vi "Set Buffer and Get Channel Reading.vi"(8 "error in":errorcluster, 9 "Readings":dbl[][](array[numeric]), 10 "Channel Ident":string, 11 "BufferLastReadingsDBL in":refnum<class "BufferLastReadsDBL.lvclass">) -> (0 "error out":errorcluster, 2 "Reading":dbl, 3 "BufferLastReadingsDBL out":refnum<class "BufferLastReadsDBL.lvclass">)   [LabVIEW 2023, in "BufferLastReadsDBL.lvclass"]
uses:
  BufferLastReadsDBL.lvclass
  BufferLastReadsDBL.lvclass/BufferLastReadsDBL.ctl
  <vilib>/Analysis/baseanly.llb/Mean (DBL).vi
  <vilib>/Analysis/NI_AALBase.lvlib
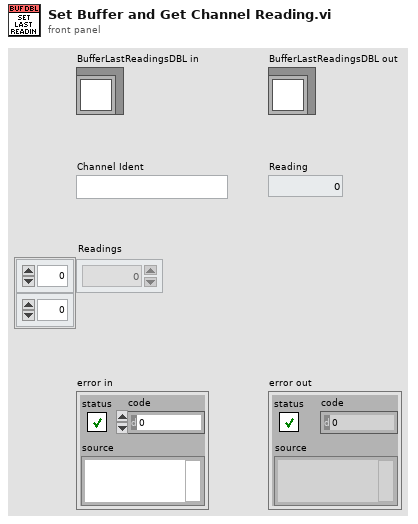
[diagram p1: front panel]
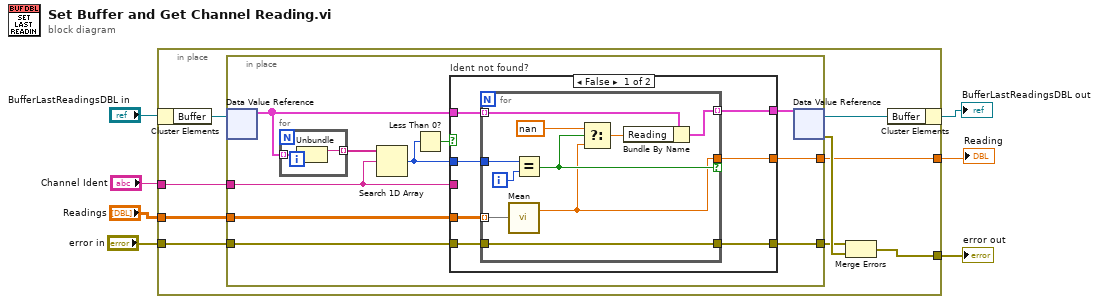
[diagram p0: block diagram]
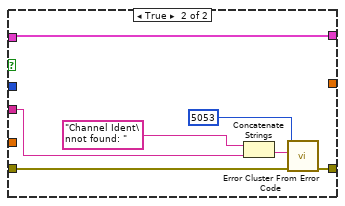
[diagram p2: hidden frame]
diagram:
  n1 = in-place {
    in-place-border: "Readings" -> [w15]
    in-place-border: "error in" -> [w14]
    in-place-border: [w12] -> w5
    in-place-border: "Channel Ident" -> [w10]
    in-place-border: [w8] -> w1
    n2 = in-place-cluster #1("BufferLastReadingsDBL in") -> ("Buffer"=w16:refnum<data-value>)
    n3 = in-place {
      in-place-border: w15 -> [w25]
      in-place-border: w14 -> [w26]
      in-place-border: w10 -> [w19]
      in-place-border: [w18] -> w9
      in-place-border: [w17] -> w8
      n4 = in-place-dvr #2(w16) -> (w21:cluster{"Ident":string, "Reading":dbl}[])  [unwired: 1 out]
      n5 = for {
        tunnel: w21 -> [w52] mode=indexing
        tunnel: [w51] -> w24 mode=indexing
        n6 = Unbundle(w52) -> ("Ident"=w51:string)  [unwired: 1 out]
      }
      n7 = Search 1D Array(1D array=w24, element=w19) -> (index of element=w22:i32)  [unwired: 1 in]
      n8 = Less Than 0?(x=w22) -> (x < 0?=w23:bool)
      n9 = case "Ident not found?" shown="False" w23 {
        tunnel: w26 -> [w28 w50]
        tunnel: w25 -> [w33 _]
        tunnel: w22 -> [w30 _]
        tunnel: w21 -> [w32 w44]
        tunnel: [w31 w44] -> w20
        tunnel: w19 -> [_ w46]
        tunnel: [w27 w45] -> w18
        tunnel: [w29 _] -> w17
        frame False {
          n10 = for {
            tunnel: w33 -> [w43] mode=indexing
            tunnel: w32 -> [w42] mode=indexing
            tunnel: [w41] -> w31 mode=indexing
            tunnel: w30 -> [w40]
            tunnel: [w35] -> w29 if=w36
            tunnel: w28 -> [w38]
            tunnel: [w38] -> w27
            i -> [w39]
            n11 = call-poly <vilib>:"Mean.vi"("X"=w43) -> ("mean"=w35:dbl)  [unwired: 1 out]
            n12 = Equal?(x=w40, y=w39) -> (x = y?=w36:bool)
            n13 = Select(t=nan, s=w36, f=w35) -> (s? t:f=w37:dbl)
            n14 = Bundle By Name(cluster=w42, "Reading"=w37) -> (w41:cluster{"Ident":string, "Reading":dbl})
          }
        }
        frame True {
          n15 = Concatenate Strings("Channel Ident\nnot found: " ("error message (\"\")"), w46) -> (w47:string)
          n16 = call <vilib>:"Error Cluster From Error Code.vi"("error in (no error)"=w50, "error message (\"\")"=w47, "error code (0)"=5053) -> ("error out"=w45:errorcluster)  [unwired: 6 in]
        }
      }
      n17 = in-place-dvr #2(w20) -> (w13:refnum<data-value>, w11:errorcluster)
    }
    n18 = Merge Errors(w9, w11) -> (w12:errorcluster)
    n19 = in-place-cluster #1("Buffer"=w13) -> (→"BufferLastReadingsDBL out":refnum<class "BufferLastReadsDBL.lvclass">)
  }
  "error out" <- w5
  "Reading" <- w1
